vi "NI6008 (volt).vi"() -> ()   [LabVIEW 2025]
panel:
  in  "created by":string
  out "volt":dbl(knob) scale=0.0..5.0
  in  "file path (use dialog)":path
  in  "stop":bool
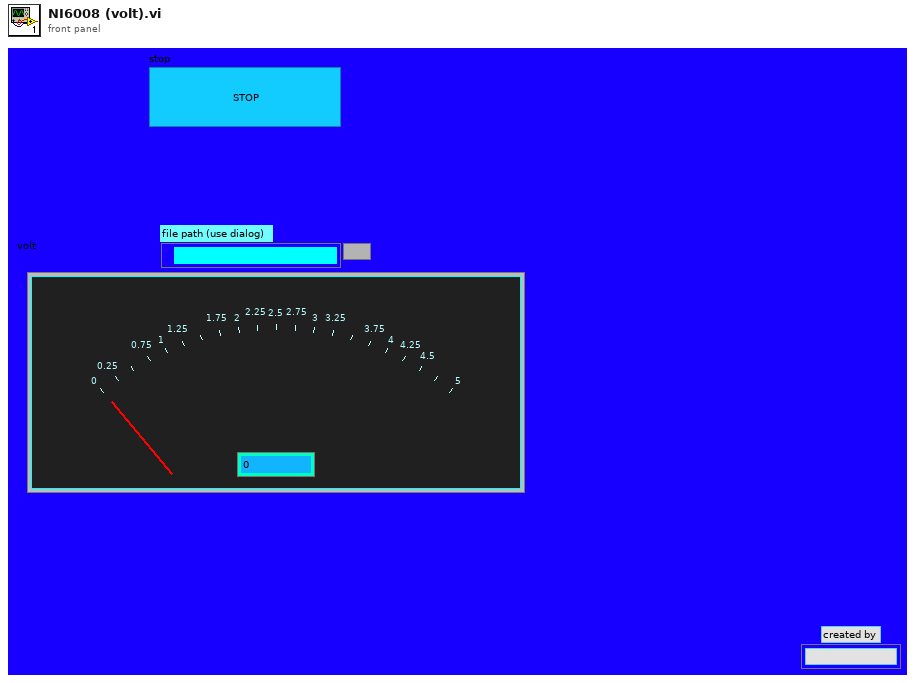
[diagram p1: front panel]
types:
  T1 = enum16{"open", "replace", "create", "open or create", "replace or create", "replace or create with confirmation"}
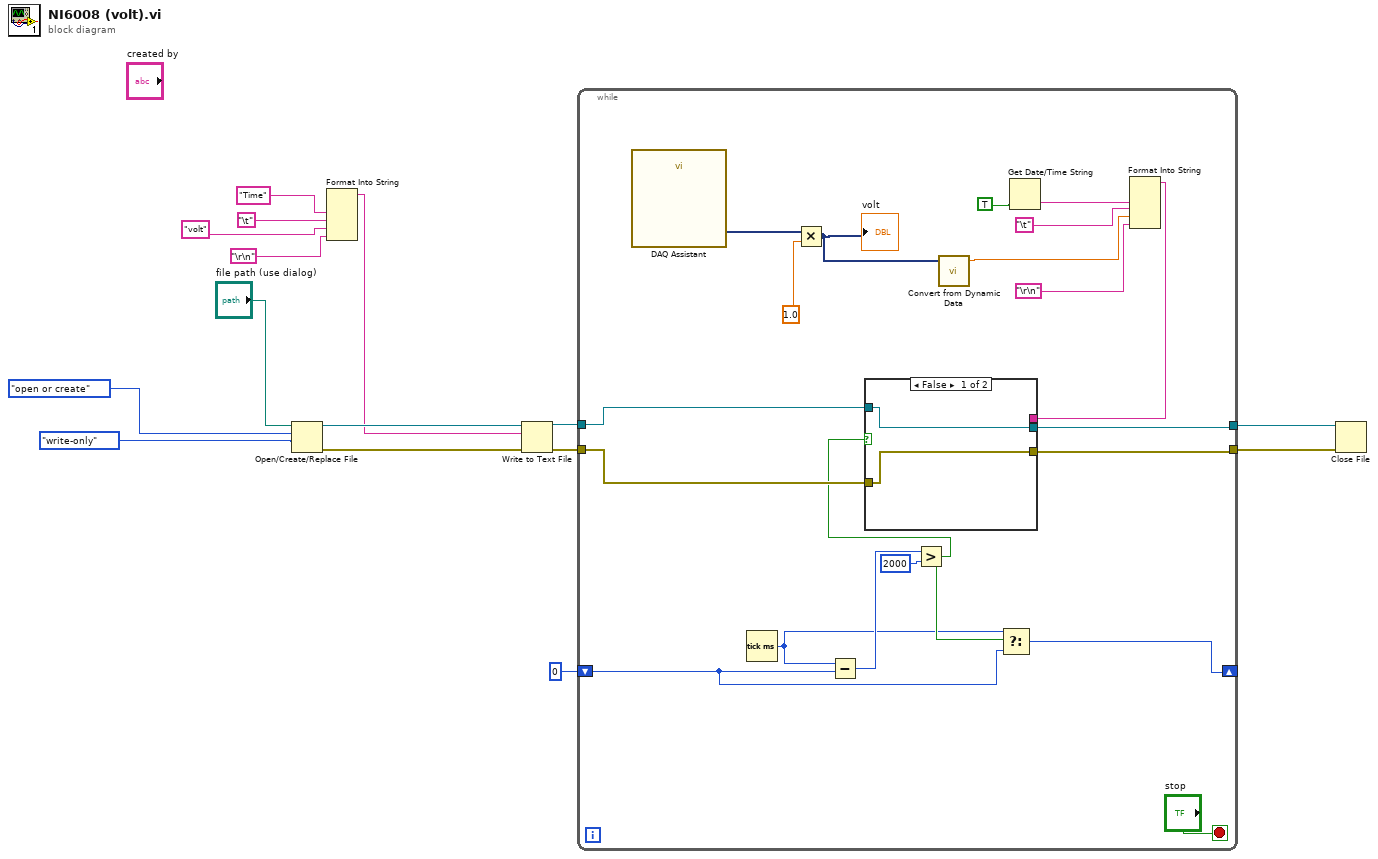
[diagram p0: block diagram]
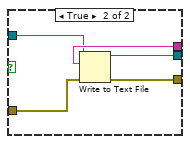
[diagram p2: hidden frame]
diagram:
  n1 = Open/Create/Replace File(file path (use dialog)="file path (use dialog)", operation (0:open)=T1."open or create", access (0:read/write)=enum16{"read/write", "read-only", "write-only"}."write-only") -> (refnum out=w5:refnum<file>, error out=w4:errorcluster)  [unwired: 3 in, 1 out]
  n2 = Format Into String("Time", "\t", "volt" ("input 6"), "\r\n") -> (resulting string=w3:string)  [unwired: 3 in, 1 out]
  n3 = Write to Text File(file (use dialog)=w5, text=w3, error in=w4) -> (refnum out=w2:refnum<file>, error out=w1:errorcluster)  [unwired: 1 in, 1 out]
  n4 = while {
    shift-right: [w20] -> _
    shift-left: 0 -> [w21]
    tunnel: [w32] -> w13
    tunnel: [w31] -> w12
    tunnel: w2 -> [w26]
    tunnel: w1 -> [w25]
    stop <- "stop" stop-if-true
    n5 = call "DAQ Assistant"() -> ("data"=w16:dynamicdata)  [unwired: 17 in, 2 out]
    n6 = Tick Count (ms)() -> (millisecond timer value=w22:u32)
    n7 = Multiply(x=w16, y=1.0) -> (x*y=w17:dynamicdata)
    "volt" <- w17
    n8 = Subtract(x=w22, y=w21) -> (x-y=w35:u32)
    n9 = Greater?(x=w35, y=2000) -> (0:w23:bool)
    n10 = call "Convert from Dynamic Data"("Dynamic Data Type"=w17) -> ("Scalar"=w27:dbl)  [unwired: 3 in]
    n11 = Select(t=w22, s=w23, f=w21) -> (s? t:f=w20:u32)
    n12 = Get Date/Time String(want seconds? (F)=TRUE) -> (time string=w30:string)  [unwired: 2 in, 1 out]
    n13 = Format Into String(w30, "\t", w27, "\r\n") -> (resulting string=w24:string)  [unwired: 3 in, 1 out]
    n14 = case shown="False" w23 {
      tunnel: [w37 w42] -> w32
      tunnel: [w36 w41] -> w31
      tunnel: w26 -> [w37 w38]
      tunnel: w25 -> [w36 w40]
      tunnel: w24 -> [_ w39]
      frame False {
      }
      frame True {
        n15 = Write to Text File(file (use dialog)=w38, text=w39, error in=w40) -> (refnum out=w42:refnum<file>, error out=w41:errorcluster)  [unwired: 1 in, 1 out]
      }
    }
  }
  n16 = Close File(refnum=w13, error in=w12) -> ()  [unwired: 2 out]
